vi "Read Sample Clipboard Q.vi"(11 "AMS Gas in":refnum<class "AMS Gas.lvclass">) -> (2 "Sample Clipboard":refnum<queue>, 3 "AMS Gas out":refnum<class "AMS Gas.lvclass">)   [LabVIEW 2015, in "AMS UI.lvlib" / "AMS Gas.lvclass"]
uses:
  AMS Gas.lvclass
  subs/Sample/Sample.lvclass
  AMS Gas.lvclass/AMS Gas.ctl
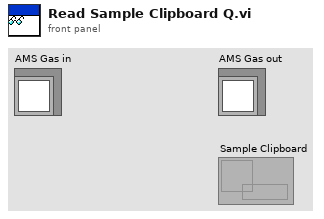
[diagram p1: front panel]
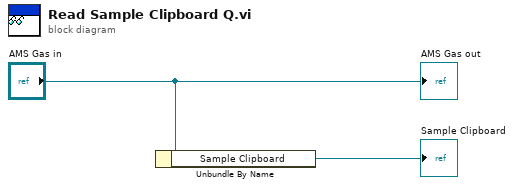
[diagram p0: block diagram]
diagram:
  n1 = Unbundle By Name("AMS Gas in") -> ("Sample Clipboard"=→"Sample Clipboard":refnum<queue>)
  "AMS Gas out" <- "AMS Gas in"
